vi "Delete State.vi"(7 "Delete Callers? (F: Only Delete Case Structure Frame)":bool, 8 "error in (no error)":errorcluster, 9 "State Name":string, 10 "Category (Optional)":string, 11 "JKI SM in":refnum<class "JKI SM.lvclass">) -> (0 "error out":errorcluster, 3 "JKI SM out":refnum<class "JKI SM.lvclass">)   [LabVIEW 2013, in "JKI State Machine API.lvlib" / "JKI SM.lvclass"]
uses:
  JKI SM.lvclass
  JKI SM.lvclass/JKI SM.ctl
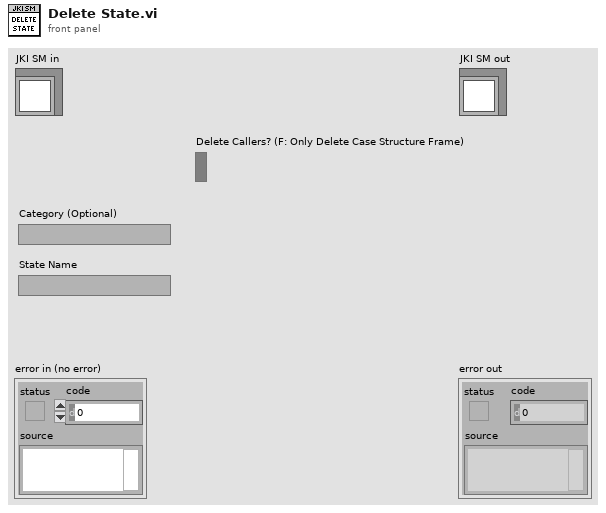
[diagram p1: front panel]
types:
  T1 = cluster{"StringConstant":refnum<vi>, "Structure":string, "Frame Name":string}[]
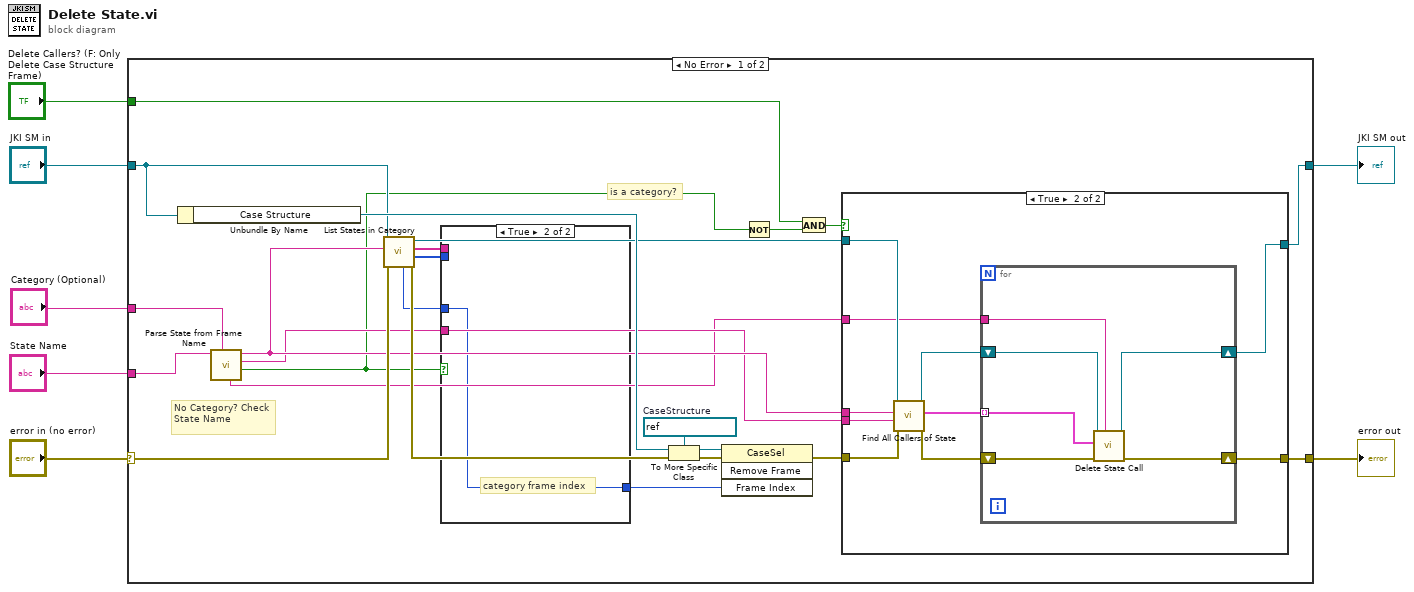
[diagram p0: block diagram]
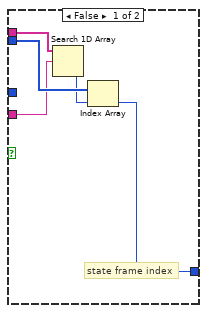
[diagram p2: hidden frame]
diagram:
  n1 = case shown="No Error" "error in (no error)" {
    selector: "error in (no error)" -> [w24 w57]
    tunnel: [w19 w57] -> w6
    tunnel: [w18 w56] -> w4
    tunnel: "JKI SM in" -> [w21 w56]
    tunnel: "State Name" -> [w16 _]
    tunnel: "Category (Optional)" -> [w17 _]
    tunnel: "Delete Callers? (F: Only Delete Case Structure Frame)" -> [w9 _]
    frame No Error {
      w29 = refnum<vi> refnum  # CaseStructure
      # "is a category?"
      # "No Category? Check State Name"
      n2 = Unbundle By Name(w21) -> ("Case Structure"=w25:refnum<vi>)
      n3 = call "Parse State from Frame Name.vi"("Category (Optional)"=w17, "Frame or State Name"=w16) -> ("is a Category Frame?"=w10:bool, "State Name"=w14:string, "Category Name"=w15:string, "\"Category: State\" String"=w13:string)  [unwired: 5 in, 1 out]
      n4 = call "List States in Category.vi"("error in (no error)"=w24, "Category"=w15, "JKI SM in"=w21) -> ("error out"=w23:errorcluster, "State Frame Indices"=w27:i32[], "States"=w28:string[], "JKI SM out"=w22:refnum<class "JKI SM.lvclass">, "Category Frame Index"=w12:i32)  [unwired: 4 in]
      n5 = case shown="True" w10 {
        tunnel: w28 -> [w36 _]
        tunnel: w27 -> [w35 _]
        tunnel: [w33 w37] -> w26
        tunnel: w14 -> [w32 _]
        tunnel: w12 -> [_ w37]
        frame False {
          # "state frame index"
          n6 = Search 1D Array(1D array=w36, element=w32) -> (index of element=w34:i32)  [unwired: 1 in]
          n7 = Index Array(array=w35, index=w34) -> (element=w33:i32)
        }
        frame True {
          # "category frame index"
        }
      }
      n8 = To More Specific Class(target class=w29, reference=w25, error in=w23) -> (specific class reference=w30:refnum<vi>, error out=w31:errorcluster)
      n9 = invoke class="CaseSel" method="Remove Frame"(reference=w30, error in=w31, "Frame Index"=w26) -> (error out=w20:errorcluster)  [unwired: 1 in, 3 out]
      n10 = Not(x=w10) -> (.not. x?=w11:bool)
      n11 = And(x=w9, y=w11) -> (x .and. y?=w8:bool)
      n12 = case shown="True" w8 {
        tunnel: w22 -> [w39 w49]
        tunnel: w20 -> [w38 w48]
        tunnel: [w38 w46] -> w19
        tunnel: [w39 w43] -> w18
        tunnel: w15 -> [_ w42]
        tunnel: w14 -> [_ w41]
        tunnel: w13 -> [_ w40]
        frame False {
        }
        frame True {
          n13 = call "Find All Callers of State.vi"("error in (no error)"=w48, "State Name"=w41, "Category (Optional)"=w42, "JKI SM in"=w49) -> ("error out"=w45:errorcluster, "Callers"=w47:T1, "JKI SM out"=w44:refnum<class "JKI SM.lvclass">)  [unwired: 5 in]
          n14 = for {
            tunnel: w47 -> [w53] mode=indexing
            shift-right: [w54] -> w46
            shift-left: w45 -> [w55]
            shift-right: [w51] -> w43
            shift-left: w44 -> [w52]
            tunnel: w40 -> [w50]
            n15 = call "Delete State Call.vi"("State"=w50, "error in (no error)"=w55, "Cluster"=w53, "JKI SM in"=w52) -> ("error out"=w54:errorcluster, "JKI SM out"=w51:refnum<class "JKI SM.lvclass">)  [unwired: 6 in]
          }
        }
      }
    }
    frame Error {
    }
  }
  "error out" <- w6
  "JKI SM out" <- w4
